vi "is valid.vi"(11 "identifying queue in":refnum<class "identifying queue.lvclass">) -> (1 "max queue size":i32, 2 "valid?":bool)   [LabVIEW 2015, in "identifying queue.lvclass"]
uses:
  identifying queue.lvclass
  identifying queue.lvclass/identifying queue.ctl
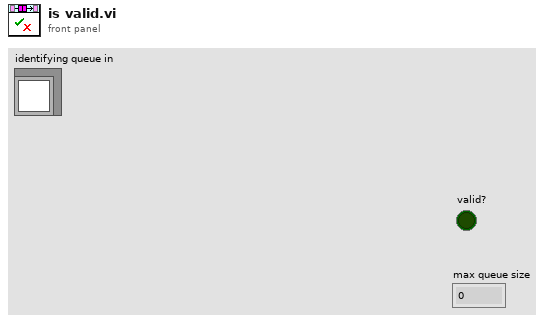
[diagram p1: front panel]
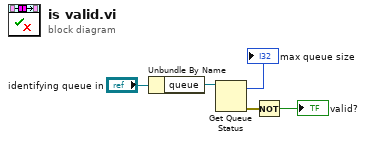
[diagram p0: block diagram]
diagram:
  n1 = Unbundle By Name("identifying queue in") -> ("queue"=w4:refnum<queue>)
  n2 = Get Queue Status(queue=w4) -> (max queue size=→"max queue size":i32, error out=w3:errorcluster)  [unwired: 2 in, 6 out]
  n3 = Not(x=w3) -> (.not. x?=→"valid?":bool)
